vi "Get Daemon Status.vi"(8 "error in (no error)":errorcluster, 11 "Modbus slave in":refnum<class "Modbus Slave.lvclass">) -> (0 "error out":errorcluster, 2 "daemon status":T1(ring), 3 "Modbus slave out":refnum<class "Modbus Slave.lvclass">)   [LabVIEW 2017, in "Modbus Slave.lvclass"]
doc: "<B>Daemon Status</B> returns the status of the daemon. A daemon has the following status: Not Started, Running, Error, and Stopped."
uses:
  <vilib>/Modbus/slave/Modbus Slave.lvclass
  <vilib>/Modbus/slave/Modbus Slave.lvclass/Modbus Slave.ctl
  <vilib>/Modbus/subvis/Protocol/Interfaces/Network Slave/Network Slave.lvclass
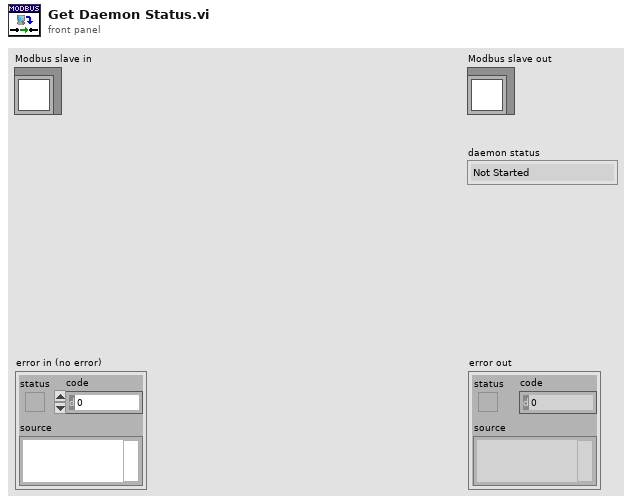
[diagram p1: front panel]
types:
  T1 = enum16{"Not Started", "Running", "Error", "Stopped"}
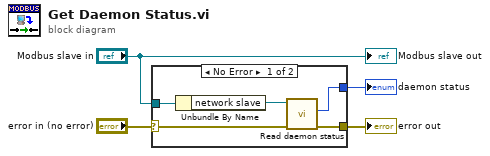
[diagram p0: block diagram]
diagram:
  n1 = case shown="No Error" "error in (no error)" {
    selector: "error in (no error)" -> [w5 w10]
    tunnel: "Modbus slave in" -> [w9 _]
    tunnel: [w7 w10] -> w3
    tunnel: [w6 _] -> w2
    frame No Error {
      n2 = Unbundle By Name(w9) -> ("network slave"=w8:refnum<class "Network Slave.lvclass">)
      n3 = call <vilib>:"Read daemon status.vi"("error in (no error)"=w5, "network slave in"=w8) -> ("error out"=w7:errorcluster, "daemon status"=w6:T1)  [unwired: 7 in, 1 out]
    }
    frame Error {
    }
  }
  "error out" <- w3
  "daemon status" <- w2
  "Modbus slave out" <- "Modbus slave in"
